vi "Read Data.vi"(4 "Source (\"\")":string, 8 "error in (no error)":errorcluster, 9 "Byte (0)":i32, 11 "VISA resource name":refnum<visa-resource-name>) -> (0 "error out":errorcluster, 1 "Read Buffer":string, 3 "VISA resource name out":refnum<visa-resource-name>)   [LabVIEW 2020, in "Yokogawa GX Series.lvlib"]
doc: "This VI reads data from the instrument."
uses:
  <instrlib>/Yokogawa GX Series/Yokogawa GX Series.lvlib
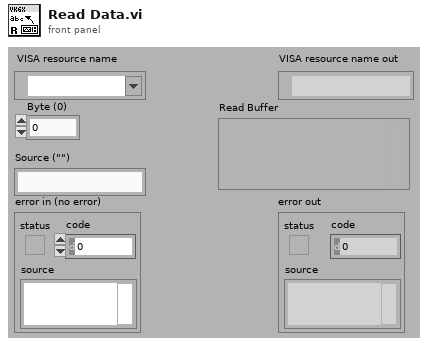
[diagram p1: front panel]
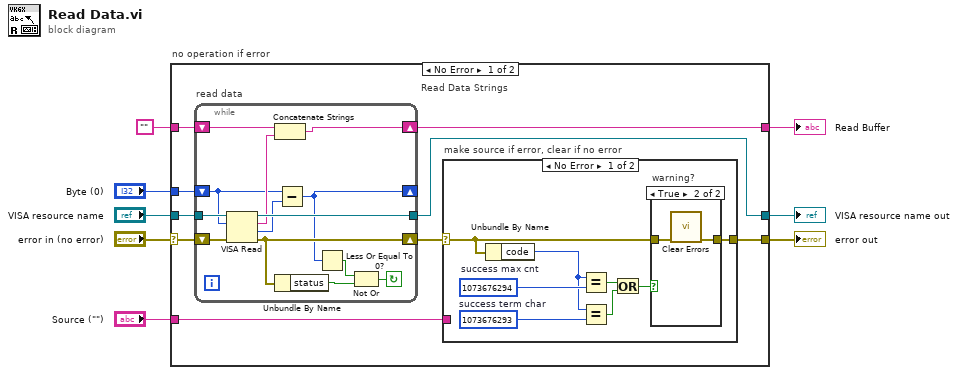
[diagram p0: block diagram]
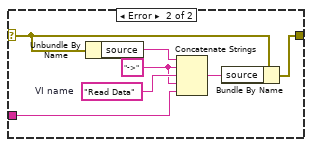
[diagram p3: hidden frame]
diagram:
  n1 = case "no operation if error" shown="No Error" "error in (no error)" {
    selector: "error in (no error)" -> [w10 w49]
    tunnel: "VISA resource name" -> [w17 w50]
    tunnel: "" -> [w16 w51]
    tunnel: [w15 w51] -> w6
    tunnel: "Byte (0)" -> [w14 _]
    tunnel: [w13 w49] -> w4
    tunnel: [w12 w50] -> w3
    tunnel: "Source (\"\")" -> [w11 _]
    frame No Error {
      # "Read Data Strings"
      n2 = while "read data" {
        shift-right: [w40] -> w9
        shift-left: w10 -> [w46]
        shift-right: [w44] -> w15
        shift-left: w16 -> [w45]
        shift-right: [w39] -> _
        shift-left: w14 -> [w42]
        tunnel: w17 -> [w48]
        tunnel: [w47] -> w12
        stop <- w36 continue-if-true
        n3 = VISA Read(VISA resource name=w48, byte count=w42, error in (no error)=w46) -> (VISA resource name out=w47:refnum<visa-resource-name>, read buffer=w43:string, return count=w41:u32, error out=w40:errorcluster)
        n4 = Concatenate Strings(w45, w43) -> (w44:string)
        n5 = Unbundle By Name(w40) -> ("status"=w37:bool)
        n6 = Subtract(x=w42, y=w41) -> (x-y=w39:u32)
        n7 = Less Or Equal To 0?(x=w39) -> (x <= 0?=w38:bool)
        n8 = Not Or(1:w37, 2:w38) -> (0:w36:bool)
      }
      n9 = case "make source if error, clear if no error" shown="No Error" w9 {
        selector: w9 -> [w18 w32]
        tunnel: [w19 w33] -> w13
        tunnel: w11 -> [_ w29]
        frame No Error {
          w24 = 1073676293  # success term char
          w25 = 1073676294  # success max cnt
          n10 = Unbundle By Name(w18) -> ("code"=w23:i32)
          n11 = Equal?(x=w23, y=w25) -> (x = y?=w22:bool)
          n12 = Equal?(x=w23, y=w24) -> (x = y?=w21:bool)
          n13 = Or(x=w22, y=w21) -> (x .or. y?=w20:bool)
          n14 = case "warning?" shown="True" w20 {
            tunnel: w18 -> [w26 w28]
            tunnel: [w26 w27] -> w19
            frame False {
            }
            frame True {
              n15 = call <vilib>:"Clear Errors.vi"("error in (no error)"=w28) -> ("error out"=w27:errorcluster)  [unwired: 1 in, 5 out]
            }
          }
        }
        frame Error {
          w31 = "Read Data"  # VI name
          w30 = "->"
          n16 = Unbundle By Name(w32) -> ("source"=w35:string)
          n17 = Concatenate Strings(w35, w30, w31, w30, w29) -> (w34:string)
          n18 = Bundle By Name(cluster=w32, "source"=w34) -> (w33:errorcluster)
        }
      }
    }
    frame Error {
    }
  }
  "VISA resource name out" <- w3
  "error out" <- w4
  "Read Buffer" <- w6
